vi "available_to_read.vi"(1 "Buffer":string) -> (0 "Available to read":u32)   [LabVIEW 2022 SP3]
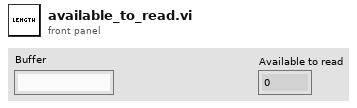
[diagram p1: front panel]
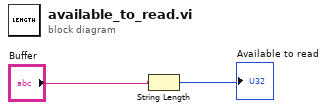
[diagram p0: block diagram]
diagram:
  n1 = String Length(string="Buffer") -> (length=→"Available to read":i32)
